vi "Trapezoid on the Fly.vi"(5 "FeedForward Constants":cluster{"kA":dbl, "kS":dbl, "kG":dbl, "kV":dbl}, 6 "Setpoint":dbl, 7 "Acceleration Max":dbl, 8 "Velocity Max":dbl, 9 "MotorControlDevRef in":T1) -> (0 "End Time":dbl, 1 "Post-Trapezoid Sensor Position":dbl, 2 "Sensor Position":dbl, 3 "MotorControlDevRef out":T1, 4 "charted V":cluster{"Sensor Velocity":dbl, "Numeric":dbl}[](array[cluster]))   [LabVIEW 2023]
uses:
  <vilib>/Rock Robotics/WPI/MotorControl/WPI_MotorControlDeviceRef.ctl
  <vilib>/Rock Robotics/WPI/MotorControl/WPI_MotorControlType.ctl
  <vilib>/Rock Robotics/SystemInterfaces/DIO/FPGA_DIOPWMChannel.ctl
  <vilib>/Rock Robotics/WPI/PWM/WPI_PWMDeadband.ctl
  <vilib>/Rock Robotics/SystemInterfaces/DIO/FPGA_DIOChannel.ctl
  <vilib>/Rock Robotics/WPI/ThirdParty/REV Robotics/REVLib/Typedef/Spark MAX Control Type.ctl
  <vilib>/Rock Robotics/WPI/ThirdParty/REV Robotics/REVLib/SubVI/Public/SPARK Get Encoder Status Position.vi
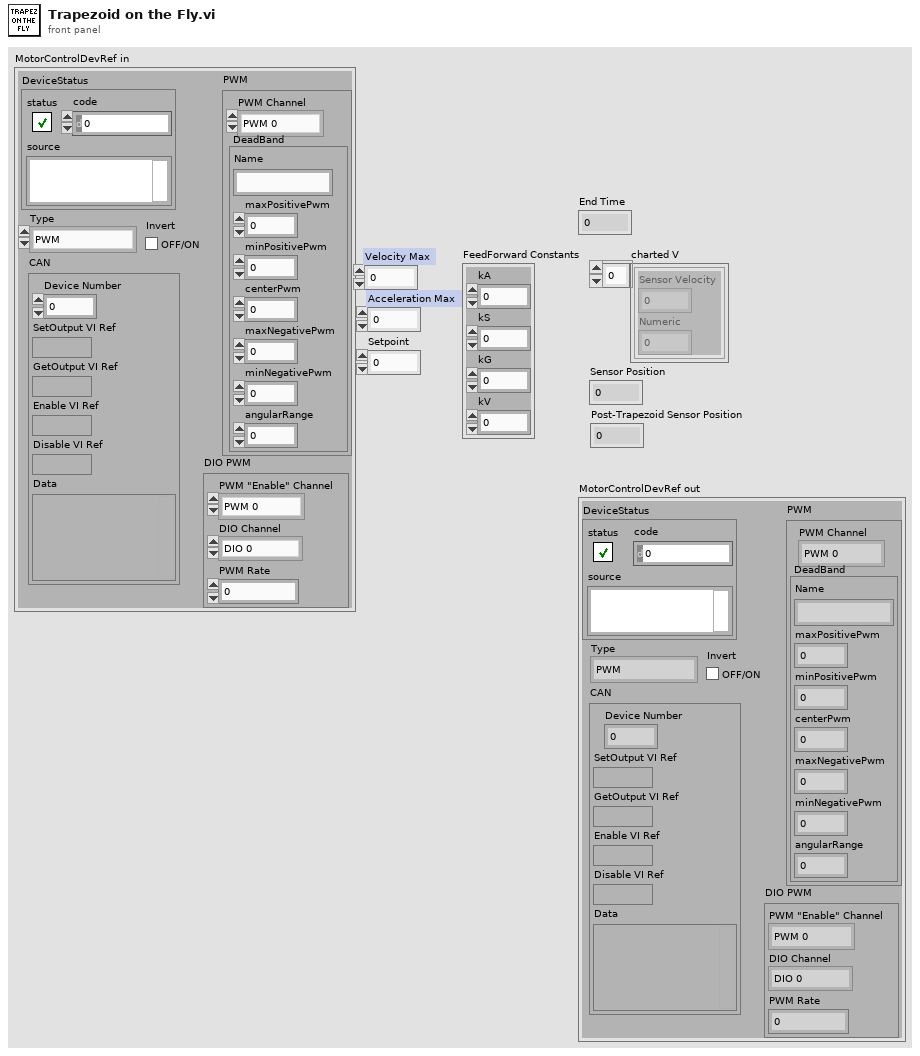
[diagram p1: front panel]
types:
  T1 = typedef "WPI_MotorControlDeviceRef.ctl" = cluster{"DeviceStatus":errorcluster, "Type":T2, "PWM":cluster{"PWM Channel":T3, "DeadBand":T4}, "CAN":cluster{"Device Number":u8, "SetOutput VI Ref":variant, "GetOutput VI Ref":variant, "Enable VI Ref":variant, "Disable VI Ref":variant, "Data":variant}, "Invert":bool, "DIO PWM":cluster{"PWM \"Enable\" Channel":T3, "DIOChannel":T5, "PWM Rate":dbl}}
  T2 = typedef "WPI_MotorControlType.ctl" = enum16{"PWM", "CAN", "DIO PWM"}
  T3 = typedef "FPGA_DIOPWMChannel.ctl" = enum8{"PWM 0", "PWM 1", "PWM 2", "PWM 3", "PWM 4", "PWM 5", "PWM 6", "PWM 7", "PWM 8", "PWM 9", "PWM MXP 0", "PWM MXP 1", "PWM MXP 2", "PWM MXP 3", "PWM MXP 4", "PWM MXP 5", "PWM MXP 6", "PWM MXP 7", "PWM MXP 8", "PWM MXP 9", "Invalid"}
  T4 = typedef "WPI_PWMDeadband.ctl" = cluster{"Name":string, "maxPositivePwm":i32, "minPositivePwm":i32, "centerPwm":i32, "maxNegativePwm":i32, "minNegativePwm":i32, "angularRange":u16}
  T5 = typedef "FPGA_DIOChannel.ctl" = enum8{"DIO 0", "DIO 1", "DIO 2", "DIO 3", "DIO 4", "DIO 5", "DIO 6", "DIO 7", "DIO 8", "DIO 9", "DIO MXP 0", "DIO MXP 1", "DIO MXP 2", "DIO MXP 3", "DIO MXP 4", "DIO MXP 5", "DIO MXP 6", "DIO MXP 7", "DIO MXP 8", "DIO MXP 9", "DIO MXP 10", "DIO MXP 11", "DIO MXP 12", "DIO MXP 13", "DIO MXP 14", "DIO MXP 15", "SPI Port CS1", "SPI Port CS2", "SPI Port CS3", "SPI Port MISO", "SPI Port MOSI", "Invalid"}
  T6 = typedef "Spark MAX Control Type.ctl" = enum16{"Percent VBus", "Voltage", "Velocity", "Position", "Smart Motion", "Current", "Smart Velocity", "MAXMotion Position", "MAXMotion Velocity"}
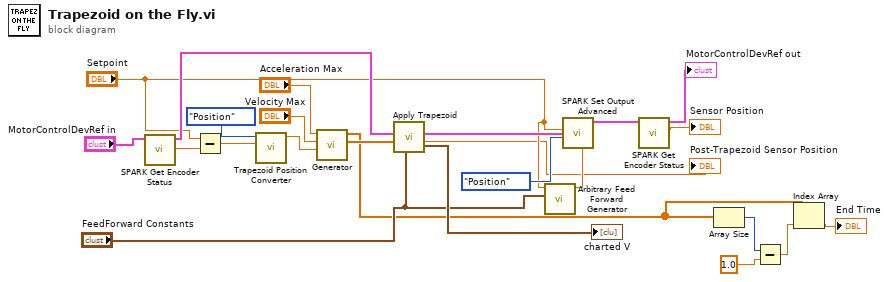
[diagram p0: block diagram]
diagram:
  n1 = call-poly <vilib>:"SPARK Get Encoder Status.vi"("MotorControlDevRef in"="MotorControlDevRef in") -> ("Sensor Position"=w12:dbl, "MotorControlDevRef out"=w18:T1)  [unwired: 7 in, 2 out]
  n2 = Subtract(x="Setpoint", y=w12) -> (x-y=w11:dbl)
  n3 = call "Trapezoid Position Converter.vi"("Distance"=w11, "Initial Parameter"=enum16{"Position", "Trapezoid Distance"}."Position") -> ("Transformed Distance"=w20:dbl)  [unwired: 9 in]
  n4 = call "Generator.vi"("Distance"=w20, "Velocity Max"="Velocity Max", "Acceleration Max"="Acceleration Max") -> ("Velocity values"=w19:dbl[], "Timestamp"=w5:dbl[])  [unwired: 7 in]
  n5 = call "Apply Trapezoid.vi"("FeedForward Constants"="FeedForward Constants", "Velocity values"=w19, "MotorControlDeviceRef in"=w18) -> ("Sensor Position"=→"Post-Trapezoid Sensor Position":dbl, "MotorControlDevRef out"=w16:T1, "charted V"=→"charted V":cluster{"Sensor Velocity":dbl, "Numeric":dbl}[])  [unwired: 5 in, 1 out]
  n6 = call "Arbitrary Feed Forward Generator.vi"("Feed Forward Constants"="FeedForward Constants", "Setpoint"="Setpoint") -> ("Arbitrary Feedforward"=w13:dbl)  [unwired: 9 in]
  n7 = call <vilib>:"SPARK Set Output Advanced.vi"("Arbitrary Feed Forward (0)"=w13, "Control Mode"=Spark_MAX_Control_Type."Position", "Setpoint"="Setpoint", "MotorControlDevRef"=w16) -> ("MotorControlDevRef"=w9:T1)  [unwired: 6 in, 1 out]
  n8 = call-poly <vilib>:"SPARK Get Encoder Status.vi"("MotorControlDevRef in"=w9) -> ("Sensor Position"=→"Sensor Position":dbl, "MotorControlDevRef out"=→"MotorControlDevRef out":T1)  [unwired: 7 in, 2 out]
  n9 = Array Size(array=w5) -> (size(s)=w2:i32)
  n10 = Subtract(x=w2, y=1.0) -> (x-y=w4:dbl)
  n11 = Index Array(array=w5, index=w4) -> (element=→"End Time":dbl)
